vi "Progress.vi"() -> ()   [LabVIEW 2019, in "PostgreSQL.lvlib"]
uses:
  PostgreSQL.lvlib
panel:
  out "DO progress":i32(slide) scale=0.0..100.0
  out "AO progress":i32(slide) scale=0.0..100.0
  out "PAR progress":i32(slide) scale=0.0..100.0
  out "ALR progress":i32(slide) scale=0.0..100.0
  out "DI progress":i32(slide) scale=0.0..100.0
  out "AI progress":i32(slide) scale=0.0..100.0
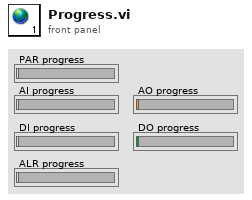
[diagram p1: front panel]
diagram:
